vi "1st order filter-LP.vi"(4 "Filter Time Constant":dbl, 6 "Dt":dbl, 8 "error in":errorcluster, 11 "Data in":dbl) -> (0 "error out":errorcluster, 3 "LP data":dbl)   [LabVIEW 2014]
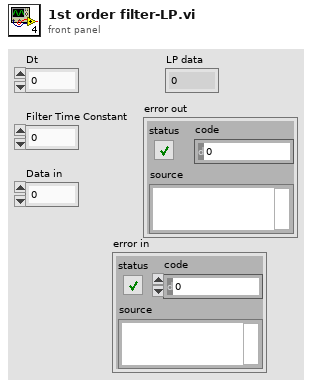
[diagram p1: front panel]
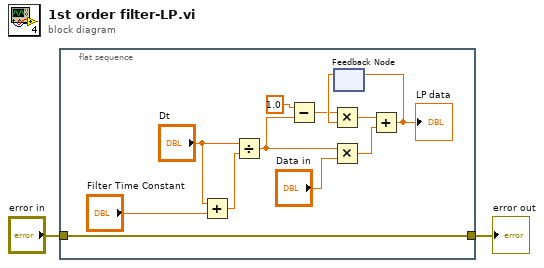
[diagram p0: block diagram]
diagram:
  n1 = flat-sequence {
    tunnel: "error in" -> [w3]
    tunnel: [w3] -> w1
    frame #0 {
      n2 = Add(x="Dt", y="Filter Time Constant") -> (x+y=w14:dbl)
      n3 = Divide(x="Dt", y=w14) -> (x/y=w9:dbl)
      n4 = Subtract(x=1.0, y=w9) -> (x-y=w5:dbl)
      n5 = Multiply(x=w9, y="Data in") -> (x*y=w10:dbl)
      n6 = feedback #1() -> (w6:dbl)  [unwired: 1 in]
      n7 = Multiply(x=w5, y=w6) -> (x*y=w7:dbl)
      n8 = Add(x=w7, y=w10) -> (x+y=w8:dbl)
      "LP data" <- w8
      n9 = feedback-in #1(w8) -> ()
    }
  }
  "error out" <- w1
